vi "ex_enableDisableItems.vi"(1 "[Refs]":refnum<vi>[](array[refnum]), 2 "Item":i32) -> (0 "Item Out":i32)   [LabVIEW 2020]
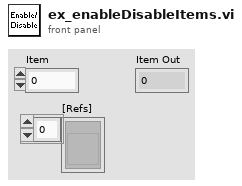
[diagram p1: front panel]
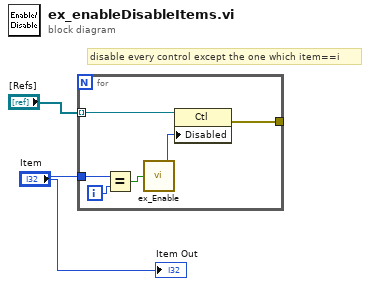
[diagram p0: block diagram]
diagram:
  # "disable every control except the one which item==i"
  n1 = for {
    tunnel: "[Refs]" -> [w8] mode=indexing
    tunnel: "Item" -> [w6]
    tunnel: [w3] -> _
    i -> [w7]
    n2 = Equal?(x=w6, y=w7) -> (x = y?=w5:bool)
    n3 = call <vilib>:"ex_Enable.vi"("Enable?"=w5) -> ("Disabled Value"=w4:u8)
    n4 = property class="Ctl"(reference=w8, "Disabled"=w4) -> (error out=w3:errorcluster)  [unwired: 1 in, 1 out]
  }
  "Item Out" <- "Item"
